vi "fifo2file.vi"(11 "DataLoggingParam":T1={"Fifo Size"=0, "FileRefnum"=refnum, "FifoRefnum"=refnum, "Fifo Time Out (ms)"=500, "MaxNumFileWrite"=255, "Force Num Array"=0}) -> (1 "fifo full counter":u16, 3 "DataLoggingParam 2":T1={"Fifo Size"=0, "FileRefnum"=refnum, "FifoRefnum"=refnum, "Fifo Time Out (ms)"=500, "MaxNumFileWrite"=255, "Force Num Array"=0}, 4 "# elements":u32)   [LabVIEW 2018, in "kevLib2010.lvlib"]
uses:
  kevLib2010.lvlib
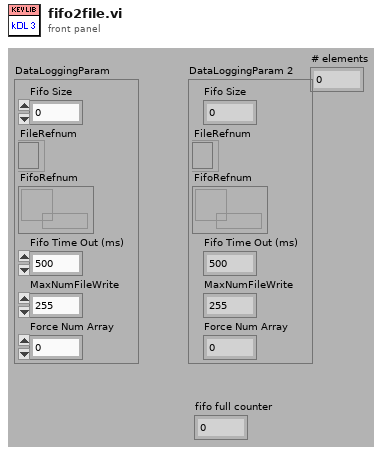
[diagram p1: front panel]
types:
  T1 = cluster{"Fifo Size":u32, "FileRefnum":refnum<file>, "FifoRefnum":refnum<k33>, "Fifo Time Out (ms)":i32, "MaxNumFileWrite":i32, "Force Num Array":i32}
  T2 = enum16{"big-endian, network order", "native, host order", "little-endian"}
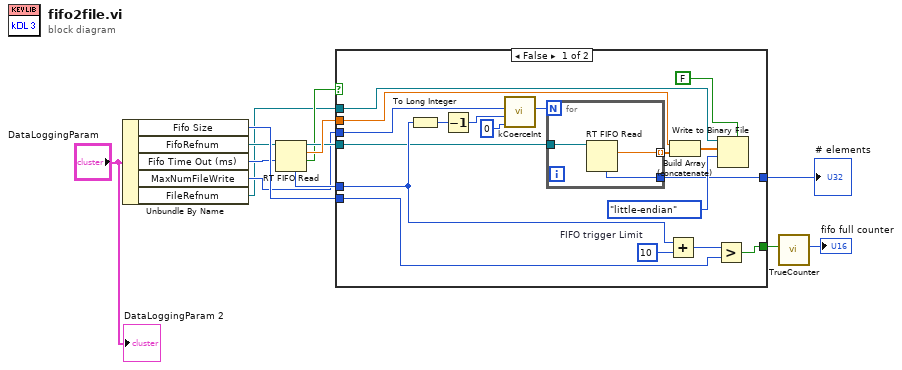
[diagram p0: block diagram]
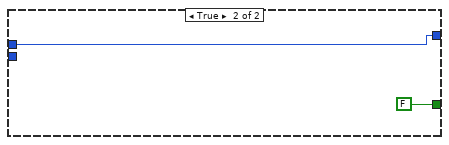
[diagram p2: hidden frame]
diagram:
  n1 = Unbundle By Name("DataLoggingParam") -> ("Fifo Size"=w6:u32, "FifoRefnum"=w5:refnum<k33>, "Fifo Time Out (ms)"=w4:i32, "MaxNumFileWrite"=w3:i32, "FileRefnum"=w2:refnum<file>)
  n2 = RT FIFO Read(0:w5, 2:w4) -> (7:w13:u32, 8:w11:refnum<k33>, 9:w12:dbl, 10:w10:bool)  [unwired: 2 in, 1 out]
  n3 = case shown="False" w10 {
    tunnel: [w31 FALSE] -> w8
    tunnel: w13 -> [w28 w35]
    tunnel: w12 -> [w25 _]
    tunnel: w11 -> [w24 _]
    tunnel: w6 -> [w17 _]
    tunnel: w3 -> [w16 _]
    tunnel: w2 -> [w15 _]
    tunnel: [w14 w35] -> w1
    frame False {
      w29 = u32 10  # FIFO trigger Limit
      n4 = To Long Integer(number=w28) -> (32bit integer=w21:i32)
      n5 = Decrement(x=w21) -> (x-1=w20:i32)
      n6 = call "kCoerceInt.vi"("lower"=0 ("lower limit"), "input"=w20, "upper"=w16) -> ("output"=w18:i32)  [unwired: 7 in, 1 out]
      n7 = for {
        N: w18 -> [_]
        tunnel: w24 -> [w34]
        tunnel: [w33] -> w26 mode=indexing
        tunnel: [w32] -> w14
        n8 = RT FIFO Read(0:w34) -> (7:w32:u32, 9:w33:dbl)  [unwired: 2 in, 4 out]
      }
      n9 = Add(x=w28, y=w29) -> (x+y=w30:u32)
      n10 = Build Array (concatenate)(w25, w26) -> (w27:dbl[])
      n11 = Greater?(x=w30, y=w17) -> (0:w31:bool)
      n12 = Write to Binary File(file (use dialog)=w15, data=w27, 5:FALSE ("prepend array or string size? (T)"), 9:T2."little-endian" ("byte order (0:big-endian, network order)")) -> ()  [unwired: 1 in, 4 out]
    }
    frame True {
    }
  }
  "# elements" <- w1
  n13 = call "TrueCounter.vi"("True?"=w8) -> ("True Count"=→"fifo full counter":u16)  [unwired: 9 in]
  "DataLoggingParam 2" <- "DataLoggingParam"
